vi "CMN_ReadCfgFromMem.vi"(0 "Vi name":string, 5 "Control Name":string, 7 "Type":string, 11 "error in":errorcluster) -> (4 "Value":string, 15 "error out":errorcluster)   [LabVIEW 2016]
panel:
  in  "Types":string[](array[string])=["STR", "BOOL", "EXT", "DBL", "SGL", "I32", "I16", "I8", "U32", "U16", "U8", "FGEnum", "PATH", "U64", "I64"]
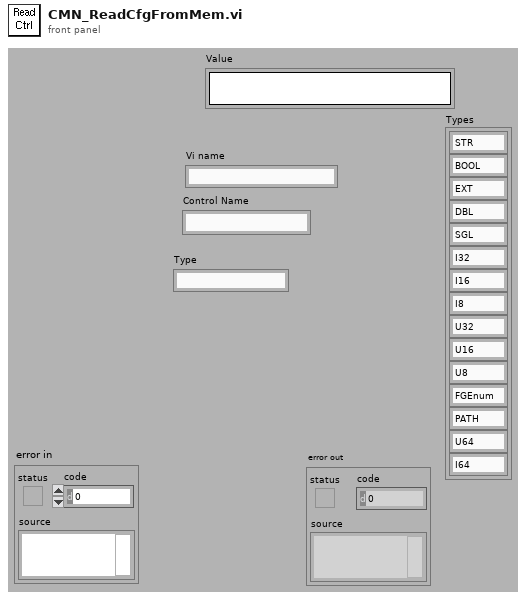
[diagram p1: front panel]
types:
  T1 = enum32{"Setup", "Settings", "Memory", "Utility", "Imaging", "Errors & Messages"}
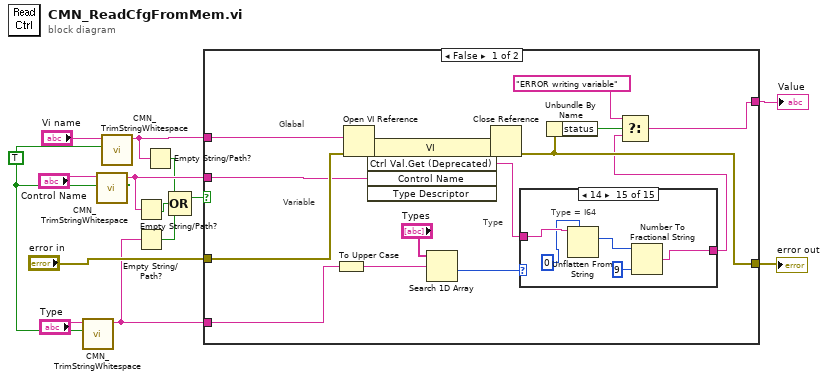
[diagram p0: block diagram]
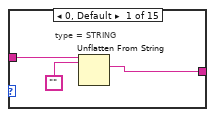
[diagram p2: hidden frame]
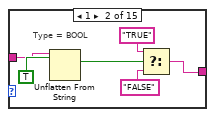
[diagram p3: hidden frame]
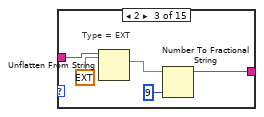
[diagram p4: hidden frame]
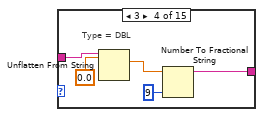
[diagram p5: hidden frame]
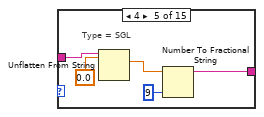
[diagram p6: hidden frame]
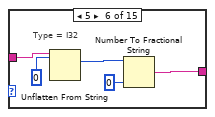
[diagram p7: hidden frame]
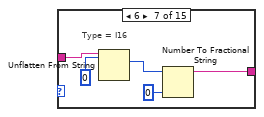
[diagram p8: hidden frame]
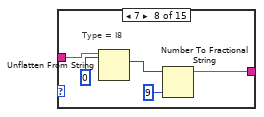
[diagram p9: hidden frame]
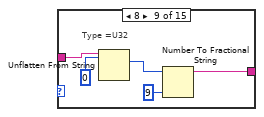
[diagram p10: hidden frame]
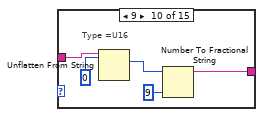
[diagram p11: hidden frame]
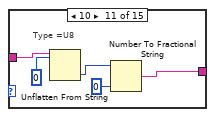
[diagram p12: hidden frame]
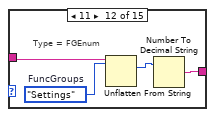
[diagram p13: hidden frame]
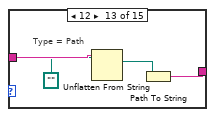
[diagram p14: hidden frame]
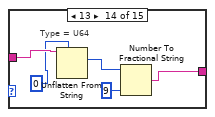
[diagram p15: hidden frame]
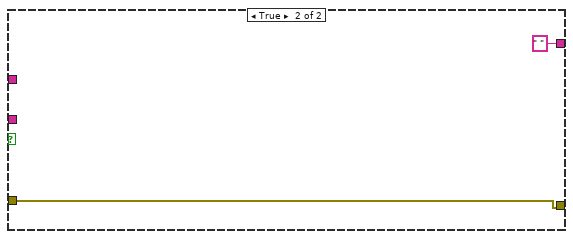
[diagram p16: hidden frame]
diagram:
  w8 = TRUE
  n1 = call "CMN_TrimStringWhitespace.vi"("Both Ends?(T)"=w8, "string"="Type") -> ("trimmed string"=w5:string)  [unwired: 8 out]
  n2 = call "CMN_TrimStringWhitespace.vi"("Both Ends?(T)"=w8, "string"="Control Name") -> ("trimmed string"=w6:string)  [unwired: 8 out]
  n3 = call "CMN_TrimStringWhitespace.vi"("Both Ends?(T)"=w8, "string"="Vi name") -> ("trimmed string"=w7:string)  [unwired: 8 out]
  n4 = Empty String/Path?(string/path=w6) -> (empty?=w3:bool)
  n5 = Empty String/Path?(string/path=w5) -> (empty?=w4:bool)
  n6 = Empty String/Path?(string/path=w7) -> (empty?=w2:bool)
  n7 = Compound Arithmetic op=OR(w2, w3, w4) -> (w1:bool)
  n8 = case shown="False" w1 {
    tunnel: [w31 w105] -> w14
    tunnel: [w30 " "] -> w13
    tunnel: "error in" -> [w29 w105]
    tunnel: w7 -> [w18 _]
    tunnel: w6 -> [w17 _]
    tunnel: w5 -> [w16 _]
    frame False {
      # "Type"
      # "Variable"
      # "Glabal"
      n9 = To Upper Case(1:w16) -> (0:w15:string)
      n10 = Open VI Reference(vi path=w18, error in (no error)=w29) -> (vi reference=w27:refnum<vi>, error out=w28:errorcluster)  [unwired: 4 out]
      n11 = invoke class="VI" method="Ctrl Val.Get (Deprecated)"(reference=w27, error in=w28, "Control Name"=w17) -> (reference out=w25:refnum<vi>, error out=w26:errorcluster, "Get Control Value"=w24:string)  [unwired: 2 in, 2 out]
      n12 = Search 1D Array(1D array="Types", element=w15) -> (index of element=w23:i32)  [unwired: 1 out]
      n13 = Close Reference(reference=w25, error in (no error)=w26) -> (error out=w31:errorcluster)
      n14 = case shown="14" w23 {
        tunnel: w24 -> [w33 w39 w44 w49 w54 w59 w64 w69 w74 w79 w84 w89 w93 w96 w101]
        tunnel: [w32 w35 w41 w46 w51 w57 w61 w66 w71 w76 w82 w87 w90 w94 w99] -> w21
        frame 0, Default {
          # "type = STRING"
          n15 = Unflatten From String(type="", binary string=w33) -> (value=w32:string)  [unwired: 1 in, 4 out]
        }
        frame 1 {
          # "Type = BOOL"
          n16 = Unflatten From String(type=TRUE, binary string=w39) -> (value=w38:bool)  [unwired: 1 in, 4 out]
          n17 = Select(t="TRUE", s=w38, f="FALSE") -> (s? t:f=w35:string)
        }
        frame 2 {
          # "Type = EXT"
          n18 = Unflatten From String(type=ext 0.0, binary string=w44) -> (value=w43:ext)  [unwired: 1 in, 4 out]
          n19 = Number To Fractional String(number=w43, precision (6)=i16 9) -> (F-format string=w41:string)  [unwired: 2 out]
        }
        frame 3 {
          # "Type = DBL"
          n20 = Unflatten From String(type=0.0, binary string=w49) -> (value=w48:dbl)  [unwired: 1 in, 4 out]
          n21 = Number To Fractional String(number=w48, precision (6)=i16 9) -> (F-format string=w46:string)  [unwired: 2 out]
        }
        frame 4 {
          # "Type = SGL"
          n22 = Unflatten From String(type=sgl 0.0, binary string=w54) -> (value=w53:sgl)  [unwired: 1 in, 4 out]
          n23 = Number To Fractional String(number=w53, precision (6)=i16 9) -> (F-format string=w51:string)  [unwired: 2 out]
        }
        frame 5 {
          # "Type = I32"
          n24 = Unflatten From String(type=0, binary string=w59) -> (value=w58:i32)  [unwired: 1 in, 4 out]
          n25 = Number To Fractional String(number=w58, precision (6)=i16 0) -> (F-format string=w57:string)  [unwired: 2 out]
        }
        frame 6 {
          # "Type = I16"
          n26 = Unflatten From String(type=i16 0, binary string=w64) -> (value=w63:i16)  [unwired: 1 in, 4 out]
          n27 = Number To Fractional String(number=w63, precision (6)=i16 0) -> (F-format string=w61:string)  [unwired: 2 out]
        }
        frame 7 {
          # "Type = I8"
          n28 = Unflatten From String(type=i8 0, binary string=w69) -> (value=w68:i8)  [unwired: 1 in, 4 out]
          n29 = Number To Fractional String(number=w68, precision (6)=i16 9) -> (F-format string=w66:string)  [unwired: 2 out]
        }
        frame 8 {
          # "Type =U32"
          n30 = Unflatten From String(type=u32 0, binary string=w74) -> (value=w73:u32)  [unwired: 1 in, 4 out]
          n31 = Number To Fractional String(number=w73, precision (6)=i16 9) -> (F-format string=w71:string)  [unwired: 2 out]
        }
        frame 9 {
          # "Type =U16"
          n32 = Unflatten From String(type=u16 0, binary string=w79) -> (value=w78:u16)  [unwired: 1 in, 4 out]
          n33 = Number To Fractional String(number=w78, precision (6)=i16 9) -> (F-format string=w76:string)  [unwired: 2 out]
        }
        frame 10 {
          # "Type =U8"
          n34 = Unflatten From String(type=u8 0, binary string=w84) -> (value=w83:u8)  [unwired: 1 in, 4 out]
          n35 = Number To Fractional String(number=w83, precision (6)=i16 0) -> (F-format string=w82:string)  [unwired: 2 out]
        }
        frame 11 {
          w88 = T1."Settings"  # FuncGroups
          # "Type = FGEnum"
          n36 = Unflatten From String(type=w88, binary string=w89) -> (value=w86:T1)  [unwired: 1 in, 4 out]
          n37 = Number To Decimal String(number=w86) -> (decimal integer string=w87:string)  [unwired: 1 out]
        }
        frame 12 {
          # "Type = Path"
          n38 = Unflatten From String(type=path "", binary string=w93) -> (value=w91:path)  [unwired: 1 in, 4 out]
          n39 = Path To String(path=w91) -> (string=w90:string)
        }
        frame 13 {
          # "Type = U64"
          n40 = Unflatten From String(type=u64 0, binary string=w96) -> (value=w98:u64)  [unwired: 1 in, 4 out]
          n41 = Number To Fractional String(number=w98, precision (6)=i16 9) -> (F-format string=w94:string)  [unwired: 2 out]
        }
        frame 14 {
          # "Type = I64"
          n42 = Unflatten From String(type=i64 0, binary string=w101) -> (value=w103:i64)  [unwired: 1 in, 4 out]
          n43 = Number To Fractional String(number=w103, precision (6)=i16 9) -> (F-format string=w99:string)  [unwired: 2 out]
        }
      }
      n44 = Unbundle By Name(w31) -> ("status"=w22:bool)
      n45 = Select(t="ERROR writing variable", s=w22, f=w21) -> (s? t:f=w30:string)
    }
    frame True {
    }
  }
  "error out" <- w14
  "Value" <- w13
